vi "GetIDs.vi"(8 "error in":errorcluster, 11 "data value reference in":T2) -> (0 "error out":errorcluster, 1 "channels":i32, 2 "groups":i32, 3 "IDs":T1)   [LabVIEW 2025, in "NISE_CEF_Tests.lvlib"]
uses:
  NISE_CEF_Tests.lvlib
  Controls/IDs.ctl
  Trunk/Configuration Framework/Node/NISE_CEF_Node.lvclass
  Trunk/Configuration Framework/Node/NodeRef.ctl
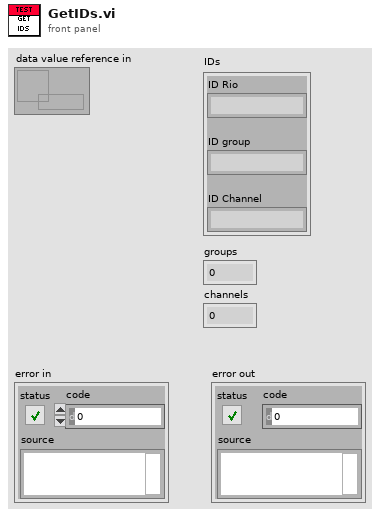
[diagram p1: front panel]
types:
  T1 = typedef "NISE_CEF_Tests.lvlib/IDs.ctl" = cluster{"ID Channel":string, "ID Rio":string, "ID group":string}
  T2 = typedef "NISE_CEF_Node.lvclass/NodeRef.ctl" = refnum<data-value>
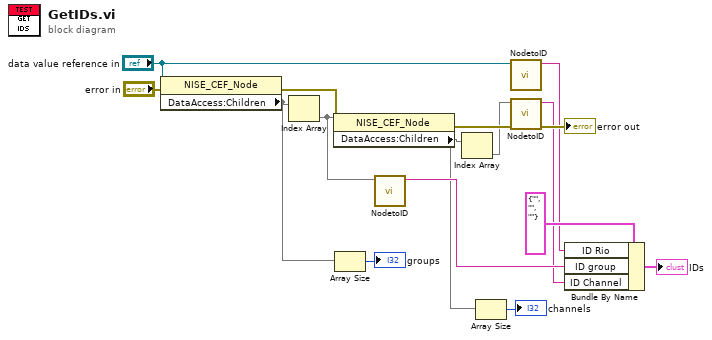
[diagram p0: block diagram]
diagram:
  n1 = property class="NISE_CEF_Node"(reference="data value reference in", error in="error in") -> (error out=w10:errorcluster, "DataAccess:Children"=w4)  [unwired: 1 out]
  n2 = Index Array(array=w4) -> (element=w14)  [unwired: 1 in]
  n3 = property class="NISE_CEF_Node"(reference=w14, error in=w10) -> (error out=w12:errorcluster, "DataAccess:Children"=w3)  [unwired: 1 out]
  n4 = Array Size(array=w4) -> (size(s)=→"groups":i32)
  n5 = call "NodetoID.vi"("node ref"=w14) -> ("ID"=w6:string)  [unwired: 9 in, 1 out]
  n6 = Index Array(array=w3) -> (element=w11)  [unwired: 1 in]
  n7 = Array Size(array=w3) -> (size(s)=→"channels":i32)
  n8 = call "NodetoID.vi"("node ref"="data value reference in") -> ("ID"=w7:string)  [unwired: 9 in, 1 out]
  n9 = call "NodetoID.vi"("error in"=w12, "node ref"=w11) -> ("error out"=→"error out":errorcluster, "ID"=w5:string)  [unwired: 8 in]
  n10 = Bundle By Name(cluster=T1 {"ID Channel"="", "ID Rio"="", "ID group"=""} ("Ids"), "ID Rio"=w7, "ID group"=w6, "ID Channel"=w5) -> (→"IDs":T1)
